vi "Parse Other Info.vi"(8 "error in (no error)":errorcluster, 10 "SR Cluster in":T1 {"Creation Date" format="%<%x>T"; "Last Updated" format="%<%x>T"}, 11 "remaining string in":string) -> (0 "error out":errorcluster, 2 "SR Cluster out 2":T1 {"Creation Date" format="%<%x>T"; "Last Updated" format="%<%x>T"}, 3 "result string":string)   [LabVIEW 2018]
uses:
  Type Defs/SR Cluster.ctl
  Type Defs/SR Status.ctl
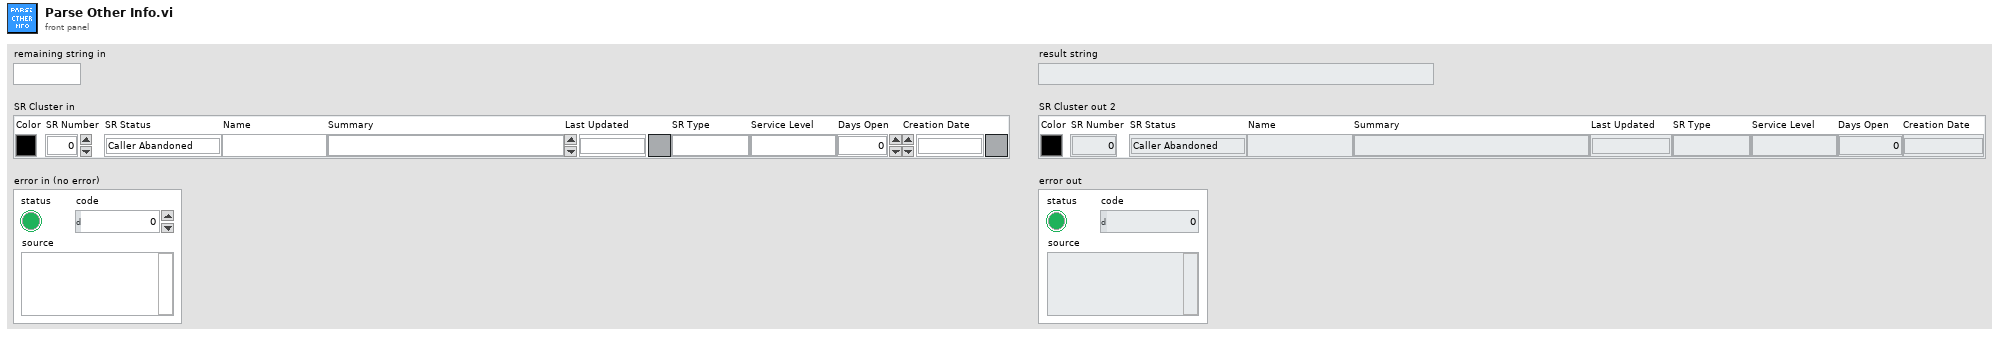
[diagram p1: front panel]
types:
  T1 = typedef "SR Cluster.ctl" = cluster{"Color":u32, "SR Number":i32, "SR Status":T2, "Name":string, "Summary":string, "Last Updated":timestamp, "SR Type":string, "Service Level":string, "Days Open":dbl, "Creation Date":timestamp}
  T2 = typedef "SR Status.ctl" = enum16{"Caller Abandoned", "Created in Error", "Expired", "Forum Resolved AE", "Forum Resolved Customer", "IN WORK", "IN WORK Collab with AES", "IN WORK Collab with PSE", "IN WORK Collab with SE", "IN WORK Customer Added Note", "IN WORK Escalation", "IN WORK Wait on Customer", "Open", "Potentially Resolved", "Presumed Resolved", "RMA Approved for Return", "Resolved", "Passed Off"}
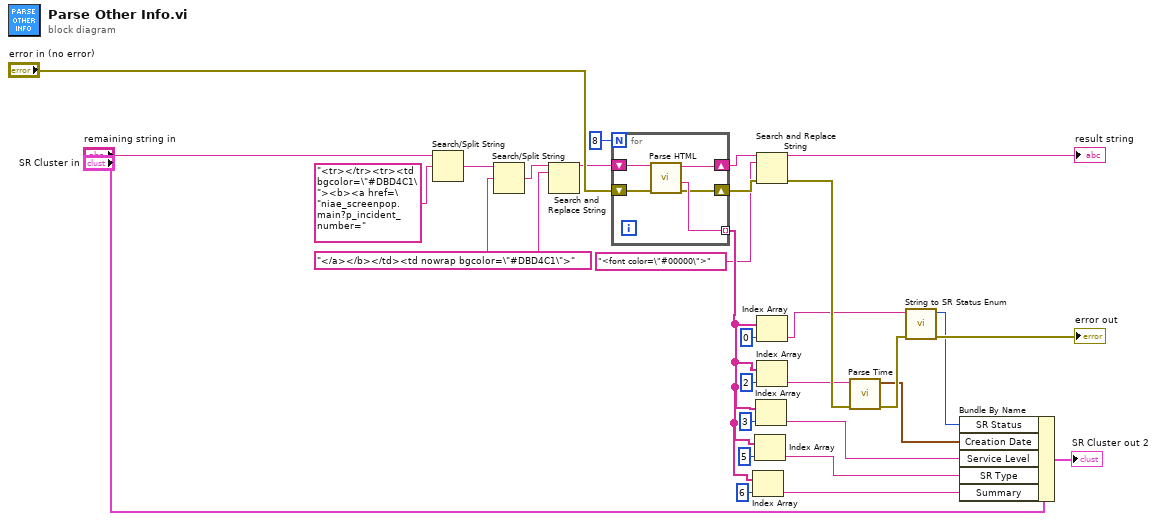
[diagram p0: block diagram]
diagram:
  w3 = "</a></b></td><td nowrap bgcolor=\"#DBD4C1\">" ("search string/char (-)")
  n1 = Search/Split String(string="remaining string in", search string/char (-)="<tr></tr><tr><td bgcolor=\"#DBD4C1\"><b><a href=\"niae_screenpop.main?p_incident_number=") -> (match + rest of string=w6:string)  [unwired: 1 in, 2 out]
  n2 = Search/Split String(string=w6, search string/char (-)=w3) -> (match + rest of string=w4:string)  [unwired: 1 in, 2 out]
  n3 = Search and Replace String(input string=w4, search string=w3) -> (result string=w2:string)  [unwired: 6 in, 3 out]
  n4 = for {
    N: 8 -> [_]
    shift-right: [w34] -> w25
    shift-left: w2 -> [w35]
    tunnel: [w33] -> w14 mode=indexing
    shift-right: [w32] -> w22
    shift-left: "error in (no error)" -> [w31]
    n5 = call "Parse HTML.vi"("error in"=w31, "result string in"=w35) -> ("error out"=w32:errorcluster, "data"=w33:string, "result string out"=w34:string)  [unwired: 7 in]
  }
  n6 = Index Array(array=w14, index=6) -> (element=w17:string)
  n7 = Index Array(array=w14, index=5) -> (element=w16:string)
  n8 = Index Array(array=w14, index=3) -> (element=w15:string)
  n9 = Search and Replace String(input string=w25, search string="<font color=\"#00000\">", error in=w22) -> (result string=→"result string":string, error out=w23:errorcluster)  [unwired: 5 in, 2 out]
  n10 = Index Array(array=w14, index=0) -> (element=w9:string)
  n11 = Index Array(array=w14, index=2) -> (element=w18:string)
  n12 = call "Parse Time.vi"("error in (no error)"=w23, "data"=w18) -> ("error out"=w27:errorcluster, "Time Stamp"=w19:timestamp)  [unwired: 8 in]
  n13 = call "String to SR Status Enum.vi"("error in"=w27, "string in"=w9) -> ("error out"=→"error out":errorcluster, "SR Status"=w10:T2)  [unwired: 8 in]
  n14 = Bundle By Name(cluster="SR Cluster in", "SR Status"=w10, "Creation Date"=w19, "Service Level"=w15, "SR Type"=w16, "Summary"=w17) -> (→"SR Cluster out 2":T1)
